vi "GPIB_663XX.vi"(1 "level (0.0 volts)":dbl caption="SET VOLT" format="%.2p", 2 "limit (0.0)":dbl caption="I LIMIT" format="%.2p", 4 "limit (22.0 volts)":dbl=22.0 caption="OVP LIMIT" format="%.2p", 5 "Output Enabled":bool, 6 "error in (no error)":errorcluster {"code" format="%.0x"}, 7 "Enum":T1(ring)=enum."Output Control", 8 "channel name (\"1\")":string="1", 9 "resource name (\"GPIB::5::INSTR\")":refnum<k15>="GPIB::5::INSTR") -> (0 "error out":errorcluster, 3 "Result":dbl)   [LabVIEW 2014]
doc: "This VI controls an Agilent GPIB Dual Power supply. The routines are:\n\nInit (initialze handle)\nSetup (set OVP, OCP, Set Voltage)\nRead Volatge\nRead Current\nOutput Control"
panel:
  out "instrument handle":refnum<k15>
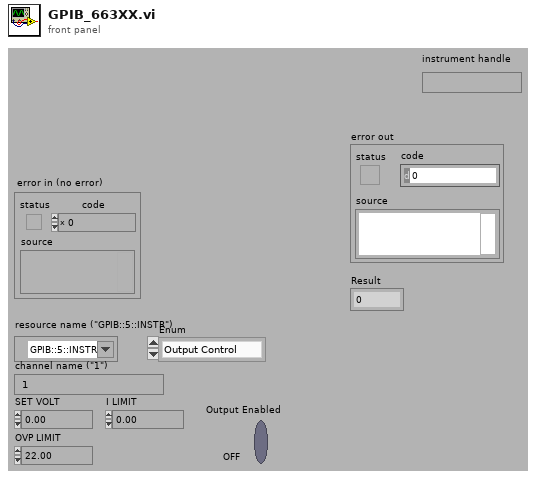
[diagram p1: front panel]
types:
  T1 = enum16{"Idle", "Init", "Setup", "Output Control", "Read Voltage", "Read Current", "DeInit Power Supply"}
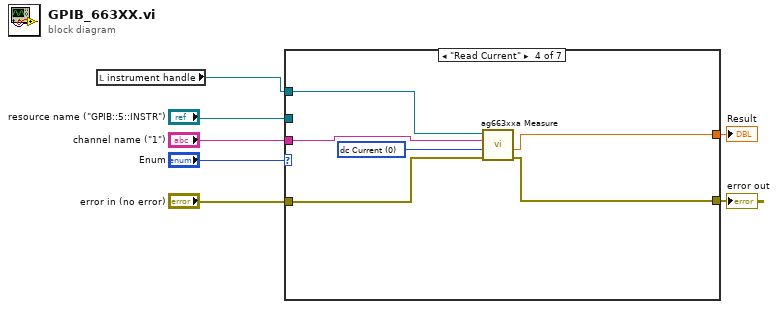
[diagram p0: block diagram]
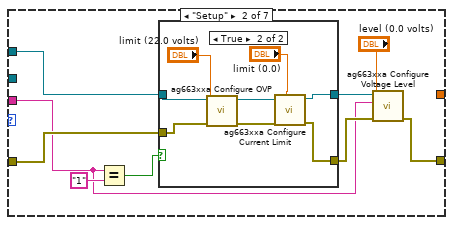
[diagram p3: hidden frame]
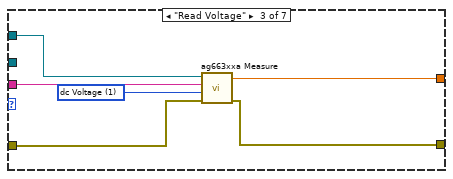
[diagram p5: hidden frame]
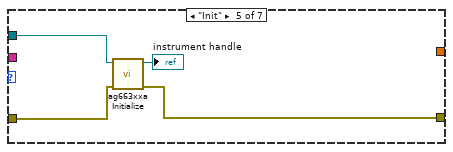
[diagram p6: hidden frame]
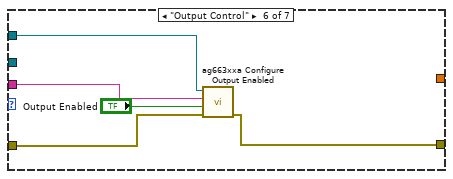
[diagram p7: hidden frame]
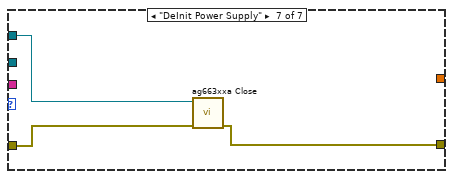
[diagram p8: hidden frame]
diagram:
  n1 = local read "instrument handle"() -> (w1:refnum<k15>)
  n2 = case shown="\"Read Current\"" "Enum" {
    tunnel: "resource name (\"GPIB::5::INSTR\")" -> [_ _ _ _ w43 _ _]
    tunnel: "error in (no error)" -> [w8 w14 w32 w37 w42 w47 w50]
    tunnel: [w8 w11 w29 w36 w41 w46 w49] -> w4
    tunnel: "channel name (\"1\")" -> [_ w10 w33 w38 _ w48 _]
    tunnel: [_ _ w31 w35 _ _ _] -> w2
    tunnel: w1 -> [_ w9 w28 w34 _ w44 w51]
    frame "Idle", Default {
    }
    frame "Setup" {
      n3 = Equal?(x=w10, y="1") -> (x = y?=w15:bool)
      n4 = case shown="True" w15 {
        tunnel: w9 -> [w18 w25]
        tunnel: [w19 w22] -> w12
        tunnel: w14 -> [w19 w21]
        tunnel: [w18 w20] -> w13
        frame False {
        }
        frame True {
          n5 = call <instrlib>:"ag663xxa Configure OVP.vi"("error in (no error)"=w21, "limit (22.0 volts)"="limit (22.0 volts)", "instrument handle"=w25) -> ("error out"=w24:errorcluster, "instrument handle out"=w23:refnum<k15>)  [unwired: 7 in]
          n6 = call <instrlib>:"ag663xxa Configure Current Limit.vi"("limit (0.0)"="limit (0.0)", "error in (no error)"=w24, "instrument handle"=w23) -> ("error out"=w22:errorcluster, "instrument handle out"=w20:refnum<k15>)  [unwired: 7 in]
        }
      }
      n7 = call <instrlib>:"ag663xxa Configure Voltage Level.vi"("error in (no error)"=w12, "level (0.0 volts)"="level (0.0 volts)", "channel name (\"1\")"=w10, "instrument handle"=w13) -> ("error out"=w11:errorcluster)  [unwired: 6 in, 1 out]
    }
    frame "Read Voltage" {
      w30 = 1 items=["dc Voltage"=1, "dc Current"=0, "ac+dc Voltage"=1001, "High Voltage Level"=1002, "Low Voltage Level"=1003, "Maximum Voltage Value"=1004, "Minimum Voltage Value"=1005, "ac+dc Current"=1006, "High Current Level"=1007, "Low Current Level"=1008, "Maximum Current Value"=1009, "Minimum Current Value"=1010] ("measurement type (1)")
      n8 = call <instrlib>:"ag663xxa Measure.vi"("error in (no error)"=w32, "measurement type (1)"=w30, "channel name (\"1\")"=w33, "instrument handle"=w28) -> ("error out"=w29:errorcluster, "measurement"=w31:dbl)  [unwired: 5 in, 1 out]
    }
    frame "Read Current" {
      w39 = 0 items=["dc Voltage"=1, "dc Current"=0, "ac+dc Voltage"=1001, "High Voltage Level"=1002, "Low Voltage Level"=1003, "Maximum Voltage Value"=1004, "Minimum Voltage Value"=1005, "ac+dc Current"=1006, "High Current Level"=1007, "Low Current Level"=1008, "Maximum Current Value"=1009, "Minimum Current Value"=1010] ("measurement type (1)")
      n9 = call <instrlib>:"ag663xxa Measure.vi"("error in (no error)"=w37, "measurement type (1)"=w39, "channel name (\"1\")"=w38, "instrument handle"=w34) -> ("error out"=w36:errorcluster, "measurement"=w35:dbl)  [unwired: 5 in, 1 out]
    }
    frame "Init" {
      n10 = call <instrlib>:"ag663xxa Initialize.vi"("error in (no error)"=w42, "resource name (\"GPIB::5::INSTR\")"=w43) -> ("error out"=w41:errorcluster, "instrument handle"=→"instrument handle":refnum<k15>)  [unwired: 8 in]
    }
    frame "Output Control" {
      n11 = call <instrlib>:"ag663xxa Configure Output Enabled.vi"("error in (no error)"=w47, "enabled (False)"="Output Enabled", "channel name (\"1\")"=w48, "instrument handle"=w44) -> ("error out"=w46:errorcluster)  [unwired: 6 in, 1 out]
    }
    frame "DeInit Power Supply" {
      n12 = call <instrlib>:"ag663xxa Close.vi"("error in (no error)"=w50, "instrument handle"=w51) -> ("error out"=w49:errorcluster)  [unwired: 9 in]
    }
  }
  "error out" <- w4
  "Result" <- w2
